vi "Process Packet.vi"(8 "error in (no error)":errorcluster, 10 "Incoming Packet":refnum<class "ControlPacket.lvclass">, 11 "Session.Client":refnum<class "Session.Client.lvclass">) -> (0 "error out":errorcluster, 3 "Session.Client":refnum<class "Session.Client.lvclass">)   [LabVIEW 2013, in "MQTT Client.lvlib" / "Session.Client.lvclass"]
uses:
  Session.Client.lvclass
  <vilib>/LabVIEW Open Source Project/MQTT Control Packets/Control Packets/ControlPacket/ControlPacket.lvclass
  MQTT_Base/Session/Session.lvclass
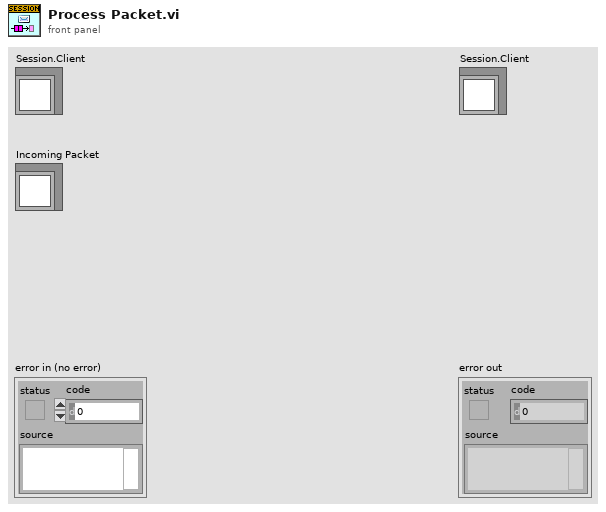
[diagram p1: front panel]
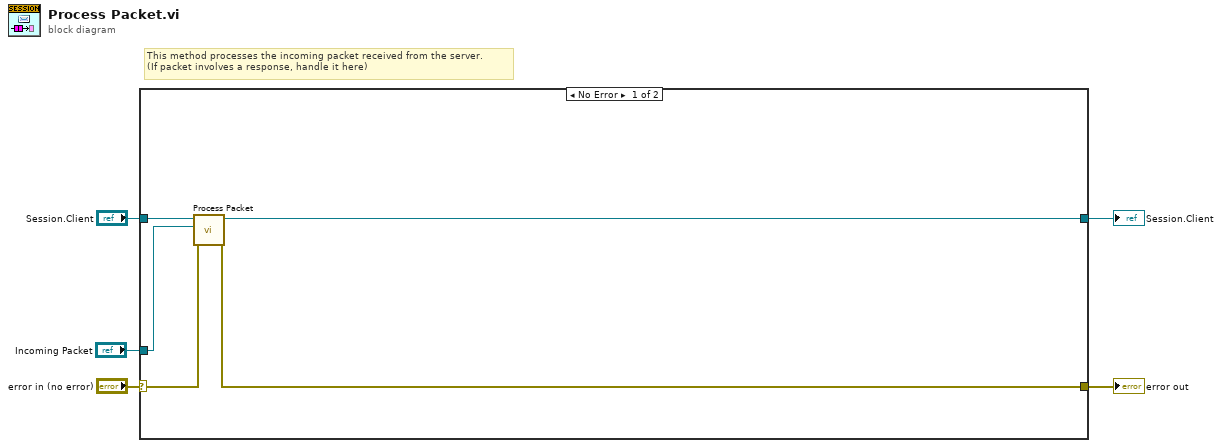
[diagram p0: block diagram]
diagram:
  # "This method processes the incoming packet received from the server.\n(If packet involves a response, handle it here)"
  n1 = case shown="No Error" "error in (no error)" {
    selector: "error in (no error)" -> [w8 w12]
    tunnel: [w6 w12] -> w4
    tunnel: [w7 w11] -> w2
    tunnel: "Session.Client" -> [w10 w11]
    tunnel: "Incoming Packet" -> [w9 _]
    frame No Error {
      n2 = call-parent "Process Packet.vi"("error in (no error)"=w8, "Incoming Packet"=w9, "Session in"=w10) -> ("error out"=w6:errorcluster, "Session out"=w7:refnum<class "Session.Client.lvclass">)  [unwired: 7 in]
    }
    frame Error {
    }
  }
  "error out" <- w4
  "Session.Client" <- w2
